vi "Osc.vi"() -> ()   [LabVIEW 2012]
uses:
  <vilib>/DAQmx/read.llb/DAQmx Read (Analog 1D Wfm NChan NSamp).vi
  <vilib>/DAQmx/create/channels.llb/DAQmx Create Channel (AI-Voltage-Basic).vi
  <vilib>/DAQmx/configure/timing.llb/DAQmx Timing (Sample Clock).vi
  <vilib>/DAQmx/configure/trigger.llb/DAQmx Start Trigger (None).vi
  <vilib>/DAQmx/miscellaneous.llb/DAQmx Fill In Error Info.vi
panel:
  in  "s":bool
  in  "stop":bool
  out "Waveform Graph":waveform(dbl)[](graph)
  in  "Timing Tab Control":enum32{""}(tab)
  in  "Timing":T1={"Sample Rate"=1000.0, "Sample Mode"=10178, "Samples per chanel"=1000, "Number of samples per channel"=-1, "Active edge"=10280} {"Active edge" items=["Rising"=10280, "Falling"=10171]; "Number of samples per channel" scale=0.0..10.0; "Samples per chanel" scale=0.0..10.0; "Sample Mode" items=["Finite Samples"=10178, "Continuous Samples"=10123, "Hardware Timed Single Point"=12522]; "Sample Rate" scale=0.0..10.0}
  in  "Channels Tab Control":enum32{"Channel A", "Channel B"}(tab)
  in  "Channel A Cluster":T2={"Maximum value "=5.0, "Minimum value"=-5.0, "Input terminal configuration "=-1, "Physical channels "=""} {"Input terminal configuration" items=["default"=-1, "RSE"=10083, "NRSE"=10078, "Differential"=10106, "Pseudodifferential"=12529]; "Minimum value" scale=0.0..10.0; "Maximum value" scale=0.0..10.0}
  in  "Channel B Cluster":T3={"Minimum value "=-5.0, "Maximum value "=5.0, "Physical channels"="", "Input terminal configuration"=-1} {"Input terminal configuration" items=["default"=-1, "RSE"=10083, "NRSE"=10078, "Differential"=10106, "Pseudodifferential"=12529]; "Maximum value" scale=0.0..10.0; "Minimum value" scale=0.0..10.0}
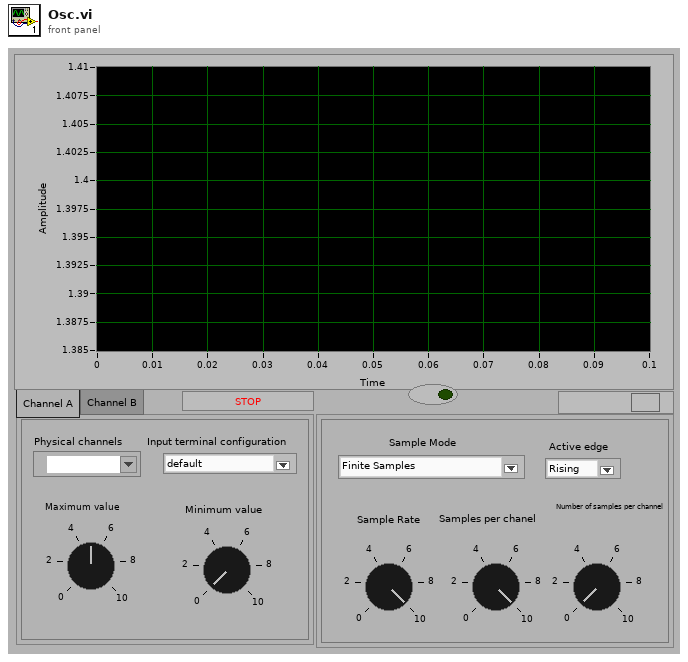
[diagram p1: front panel]
types:
  T1 = cluster{"Sample Rate":dbl, "Sample Mode":i32, "Samples per chanel":i32, "Number of samples per channel":i32, "Active edge":i32}
  T2 = cluster{"Maximum value ":dbl, "Minimum value":dbl, "Input terminal configuration ":i32, "Physical channels ":tag}
  T3 = cluster{"Minimum value ":dbl, "Maximum value ":dbl, "Physical channels":tag, "Input terminal configuration":i32}
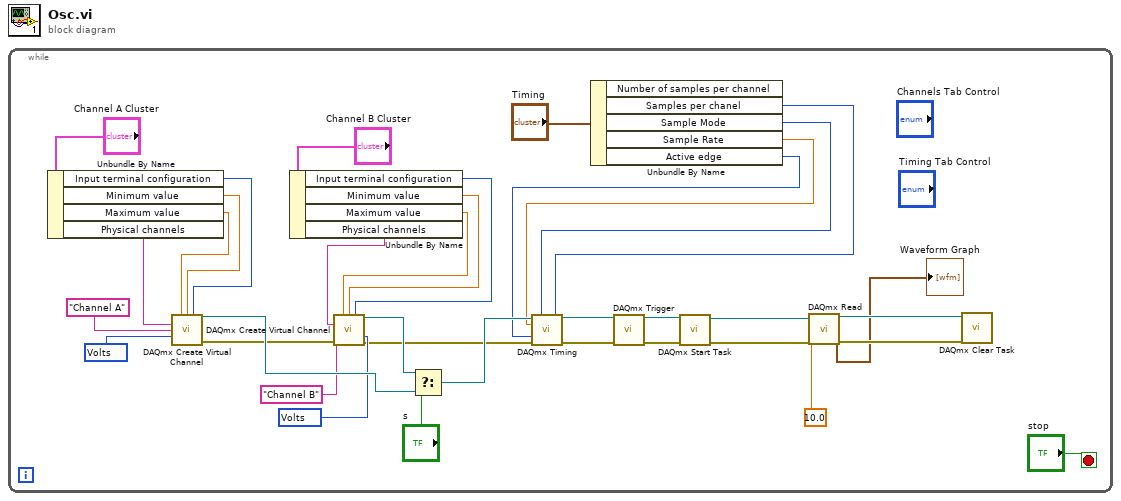
[diagram p0: block diagram]
diagram:
  n1 = while {
    stop <- "stop" stop-if-true
    w14 = 10348 items=["Volts"=10348, "From Custom Scale"=10065] ("units")
    w7 = 10348 items=["Volts"=10348, "From Custom Scale"=10065] ("units")
    n2 = Unbundle By Name("Channel A Cluster") -> ("Input terminal configuration"=w18:i32, "Minimum value"=w17:dbl, "Maximum value"=w16:dbl, "Physical channels"=w15:tag)
    n3 = call-poly <vilib>:"DAQmx Create Virtual Channel.vi"("maximum value"=w16, "minimum value"=w17, "input terminal configuration"=w18, "physical channels"=w15, "name to assign"="Channel A", "units"=w7) -> ("task out"=w30:refnum<k21>, "error out"=w10:errorcluster)  [unwired: 8 in]
    n4 = Unbundle By Name("Channel B Cluster") -> ("Input terminal configuration"=w19:i32, "Minimum value"=w22:dbl, "Maximum value"=w21:dbl, "Physical channels"=w20:tag)
    n5 = call-poly <vilib>:"DAQmx Create Virtual Channel.vi"("maximum value"=w21, "minimum value"=w22, "input terminal configuration"=w19, "physical channels"=w20, "name to assign"="Channel B", "units"=w14, "error in"=w10) -> ("task out"=w28:refnum<k21>, "error out"=w11:errorcluster)  [unwired: 7 in]
    n6 = Select(t=w28, s="s", f=w30) -> (s? t:f=w29:refnum<k21>)
    n7 = Unbundle By Name("Timing") -> ("Samples per chanel"=w25:i32, "Sample Mode"=w26:i32, "Sample Rate"=w24:dbl, "Active edge"=w27:i32)  [unwired: 1 out]
    n8 = call-poly <vilib>:"DAQmx Timing.vi"("task/channels in"=w29, "sample mode"=w26, "samples per channel"=w25, "rate"=w24, "active edge"=w27, "error in"=w11) -> ("task out"=w3:refnum<k21>, "error out"=w4:errorcluster)  [unwired: 8 in]
    n9 = call-poly <vilib>:"DAQmx Trigger.vi"("task/channels in"=w3, "error in"=w4) -> ("task out"=w6:refnum<k21>, "error out"=w5:errorcluster)  [unwired: 12 in]
    n10 = call <vilib>:"DAQmx Start Task.vi"("task/channels in"=w6, "error in"=w5) -> ("task out"=w33:refnum<k21>, "error out"=w34:errorcluster)  [unwired: 12 in]
    n11 = call-poly <vilib>:"DAQmx Read.vi"("task/channels in"=w33, "timeout"=10.0, "error in"=w34) -> ("task out"=w35:refnum<k21>, "data"=→"Waveform Graph":waveform(dbl)[], "error out"=w36:errorcluster)  [unwired: 10 in]
    n12 = call <vilib>:"DAQmx Clear Task.vi"("task in"=w35, "error in"=w36) -> ()  [unwired: 13 in, 1 out]
  }
